vi "make_current_default.vi"() -> ()   [LabVIEW 2018]
panel:
  in  "vi path":path
  # "Saving control values..."
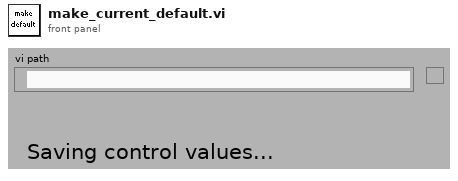
[diagram p1: front panel]
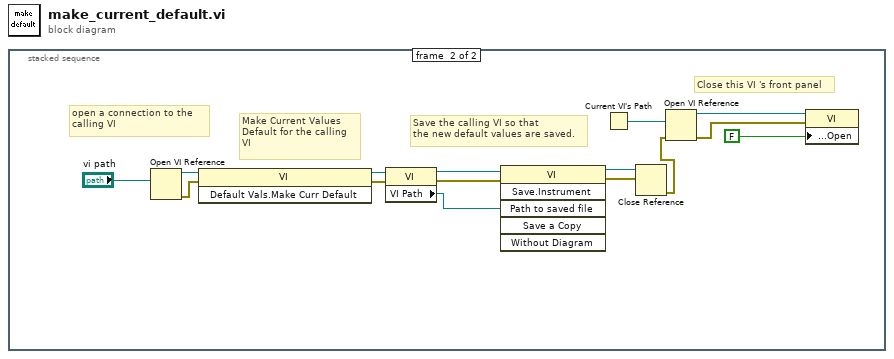
[diagram p0: block diagram]
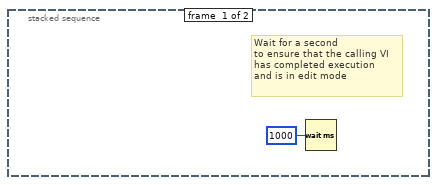
[diagram p2: hidden frame]
diagram:
  n1 = stacked-sequence {
    frame #0 {
      # "Wait for a second \nto ensure that the calling VI \nhas completed execution \nand is in edit mode"
      n2 = Wait (ms)(milliseconds to wait=u32 1000) -> ()  [unwired: 1 out]
    }
    frame #1 {
      # "Close this VI 's front panel"
      # "Save the calling VI so that\nthe new default values are saved."
      # "Make Current Values\nDefault for the calling \nVI"
      # "open a connection to the \ncalling VI"
      n3 = Open VI Reference(vi path="vi path") -> (vi reference=w13:refnum<vi>, error out=w12:errorcluster)  [unwired: 5 in]
      n4 = invoke class="VI" method="Default Vals.Make Curr Default"(reference=w13, error in=w12) -> (reference out=w11:refnum<vi>, error out=w10:errorcluster)  [unwired: 1 in, 1 out]
      n5 = property class="VI"(reference=w11, error in=w10) -> (reference out=w9:refnum<vi>, error out=w8:errorcluster, "VI Path"=w7:path)
      n6 = invoke class="VI" method="Save.Instrument"(reference=w9, error in=w8, "Path to saved file"=w7) -> (reference out=w15:refnum<vi>, error out=w14:errorcluster)  [unwired: 3 in, 4 out]
      n7 = Current VI's Path() -> (path=w6:path)
      n8 = Close Reference(reference=w15, error in (no error)=w14) -> (error out=w5:errorcluster)
      n9 = Open VI Reference(vi path=w6, error in (no error)=w5) -> (vi reference=w4:refnum<vi>, error out=w3:errorcluster)  [unwired: 4 in]
      n10 = property class="VI"(reference=w4, error in=w3, "Front Panel Window:Open"=FALSE) -> ()  [unwired: 2 out]
    }
  }
